vi "Calculate Test Parameters for Histogram.vi"(9 "test duration (sec)":dbl, 10 "input frequency":dbl, 11 "sample rate":u32) -> (0 "acquisition duration":dbl, 1 "actual number of cycles":u32, 2 "samples to acquire":u32, 3 "input frequency":dbl)   [LabVIEW 2021]
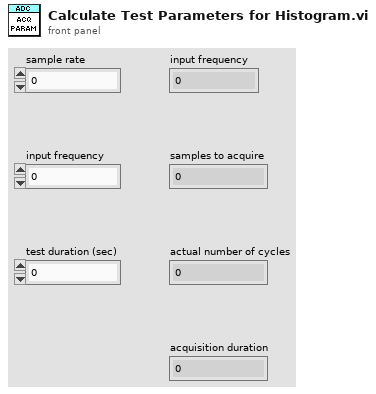
[diagram p1: front panel]
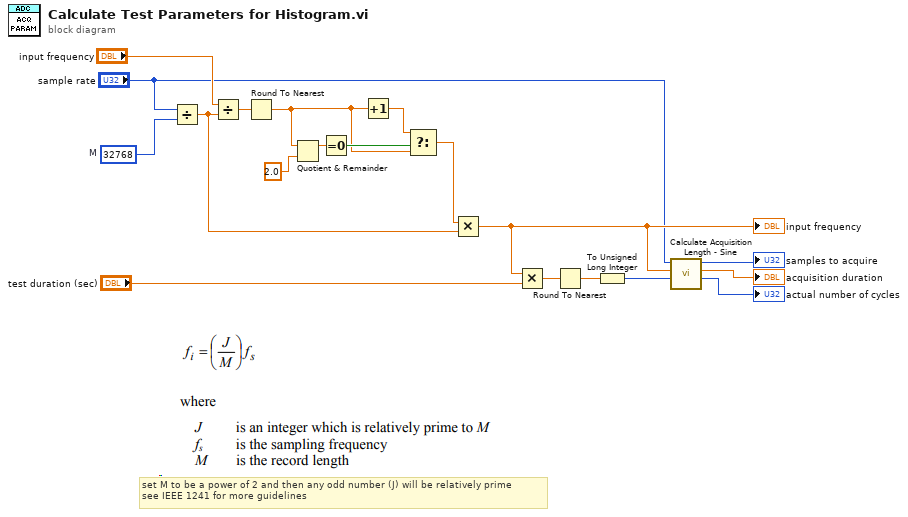
[diagram p0: block diagram]
diagram:
  w19 = 32768  # M
  # "set M to be a power of 2 and then any odd number (J) will be relatively prime\nsee IEEE 1241 for more guidelines"
  n1 = Divide(x="sample rate", y=w19) -> (x/y=w10:dbl)
  n2 = Divide(x="input frequency", y=w10) -> (x/y=w17:dbl)
  n3 = Round To Nearest(number=w17) -> (nearest integer value=w12:dbl)
  n4 = Quotient & Remainder(x=w12, y=2.0) -> (x-y*floor(x/y)=w15:dbl)  [unwired: 1 out]
  n5 = Equal To 0?(x=w15) -> (x = 0?=w14:bool)
  n6 = Increment(x=w12) -> (x+1=w13:dbl)
  n7 = Select(t=w13, s=w14, f=w12) -> (s? t:f=w11:dbl)
  n8 = Multiply(x=w11, y=w10) -> (x*y=w5:dbl)
  "input frequency" <- w5
  n9 = Multiply(x=w5, y="test duration (sec)") -> (x*y=w8:dbl)
  n10 = Round To Nearest(number=w8) -> (nearest integer value=w7:dbl)
  n11 = To Unsigned Long Integer(number=w7) -> (unsigned 32bit integer=w6:u32)
  n12 = call "Calculate Acquisition Length - Sine.vi"("number of cycles to acquire"=w6, "input frequency"=w5, "sample rate"="sample rate") -> ("actual number of cycles"=→"actual number of cycles":u32, "acquisition duration"=→"acquisition duration":dbl, "samples to acquire"=→"samples to acquire":u32)  [unwired: 6 in]
